vi "Floc Depth GUI.vi"(6 "Floc Depth r/w control":T2(ring), 8 "error in (no error)":errorcluster, 10 "HW.FlocEndDepthIntput":dbl[unit], 11 "Floc Depth Ref 2":T1) -> (0 "error out":errorcluster, 2 "HW.FlocEndDepth Output":dbl[unit])   [LabVIEW 2015, in "AguaClara Library.lvlib"]
uses:
  AguaClara Library.lvlib
  Floc Depth Ref.ctl
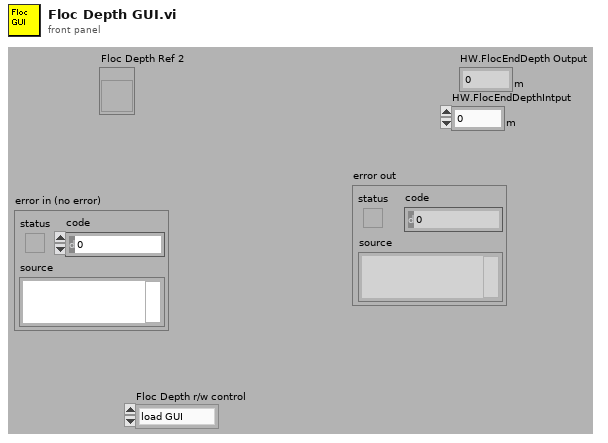
[diagram p1: front panel]
types:
  T1 = typedef "Floc Depth Ref.ctl" = refnum<vi>
  T2 = enum16{"load GUI", "write to GUI", "Update GUI", "write to basic inputs", "read from basic inputs"}
  T3 = cluster{"HW.FlocEnd":enum32{"User specified depth", "Same depth as sed tank", "Maximum depth for horizontal flow flocculator"}, "HW.FlocEndDepth":dbl[unit]}
  T4 = enum32{"User specified depth", "Same depth as sed tank", "Minimum depth for horizontal flow FLocculator"}
  T5 = enum32{"User specified depth", "Same depth as sed tank", "Maximum depth for horizontal flow flocculator"}
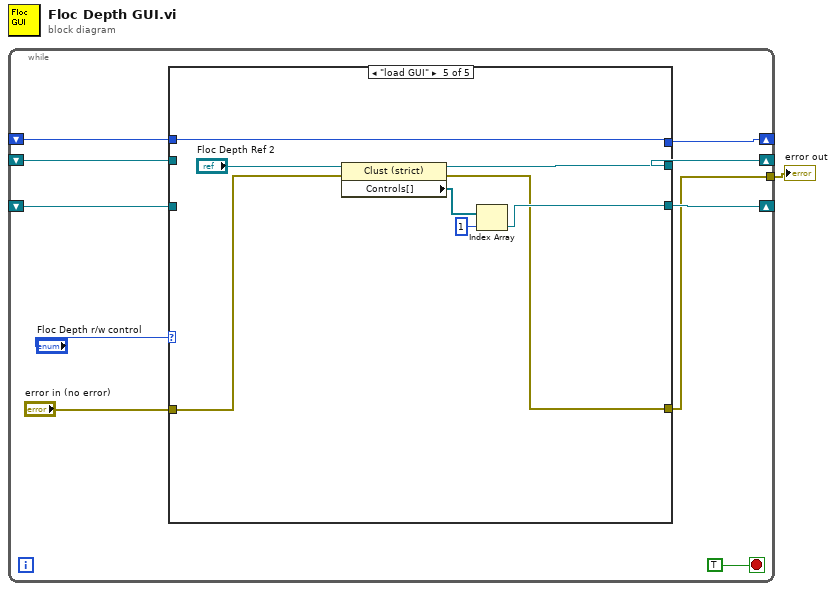
[diagram p0: block diagram]
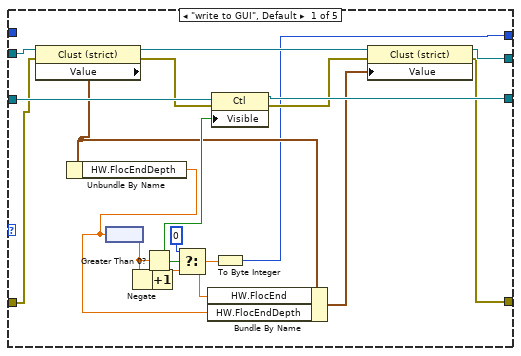
[diagram p2: hidden frame]
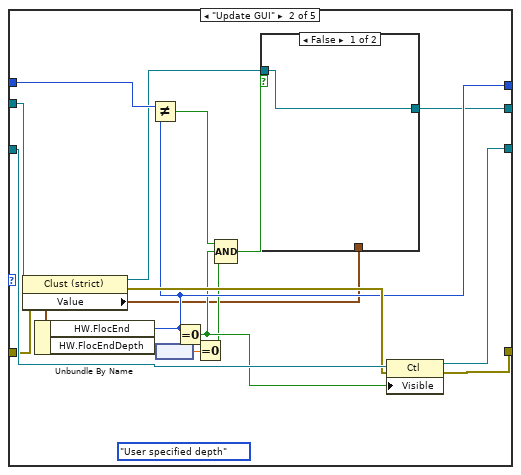
[diagram p3: hidden frame]
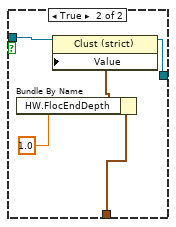
[diagram p4: hidden frame]
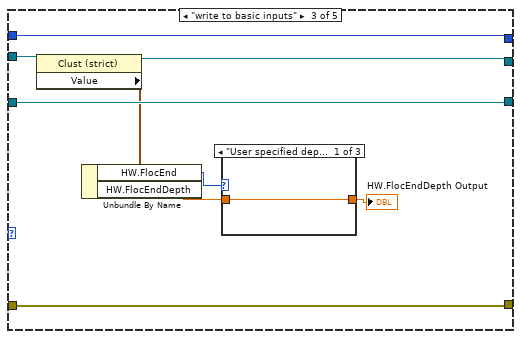
[diagram p5: hidden frame]
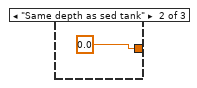
[diagram p6: hidden frame]
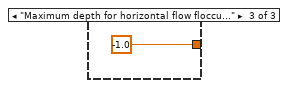
[diagram p7: hidden frame]
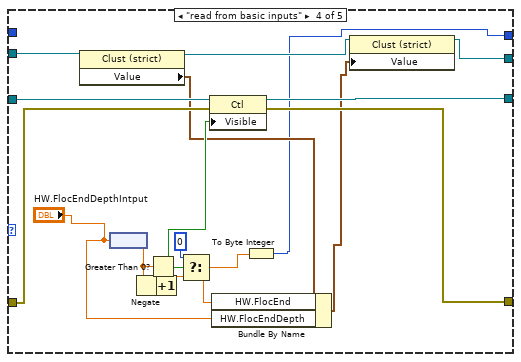
[diagram p8: hidden frame]
diagram:
  n1 = while {
    shift-right: [w9] -> _
    shift-left: _ -> [w7]
    shift-right: [w8] -> _
    shift-left: _ -> [w6]
    tunnel: [w4] -> w1
    shift-right: [w3] -> _
    shift-left: _ -> [w2]
    stop <- TRUE stop-if-true
    n2 = case shown="\"load GUI\"" "Floc Depth r/w control" {
      tunnel: w6 -> [w25 w47 w62 w76 _]
      tunnel: [w22 w31 w56 w72 w89] -> w9
      tunnel: w7 -> [w18 w44 w57 w70 _]
      tunnel: [w23 w46 w62 w75 w86] -> w8
      tunnel: [w19 w45 w61 w73 w84] -> w4
      tunnel: "error in (no error)" -> [w15 w43 w61 w74 w85]
      tunnel: [w12 w40 w54 w66 w83] -> w3
      tunnel: w2 -> [_ w41 w54 _ w83]
      frame "write to GUI", Default {
        n3 = property class="Clust (strict)"(reference=w18, error in=w15) -> (reference out=w17:T1, error out=w14:errorcluster, "Value"=w16:T3)
        n4 = Unbundle By Name(w16) -> ("HW.FlocEndDepth"=w26:dbl[unit])
        n5 = node(w26) -> (w29:dbl)
        n6 = Negate(x=w29) -> (-x=w28:dbl)
        n7 = Greater Than 0?(x=w29) -> (x > 0?=w24:bool)
        n8 = Increment(x=w28) -> (x+1=w27:dbl)
        n9 = Select(t=0, s=w24, f=w27) -> (s? t:f=w13:dbl)
        n10 = Bundle By Name(cluster=w16, "HW.FlocEnd"=w13, "HW.FlocEndDepth"=w26) -> (w21:T3)
        n11 = property class="Ctl"(reference=w25, error in=w14, "Visible"=w24) -> (reference out=w23:refnum<vi>, error out=w20:errorcluster)
        n12 = To Byte Integer(number=w13) -> (8bit integer=w12:i8)
        n13 = property class="Clust (strict)"(reference=w17, error in=w20, "Value"=w21) -> (reference out=w22:T1, error out=w19:errorcluster)
      }
      frame "Update GUI" {
        (unwired) T4."User specified depth" ("HW.FlocEnd")
        n14 = property class="Clust (strict)"(reference=w44, error in=w43) -> (reference out=w32:T1, error out=w42:errorcluster, "Value"=w33:T3)
        n15 = Unbundle By Name(w33) -> ("HW.FlocEnd"=w40:T5, "HW.FlocEndDepth"=w39:dbl[unit])
        n16 = Not Equal?(x=w41, y=w40) -> (x != y?=w37:bool)
        n17 = node(w39) -> (w38:dbl)
        n18 = Equal To 0?(x=w40) -> (x = 0?=w36:bool)
        n19 = Equal To 0?(x=w38) -> (x = 0?=w35:bool)
        n20 = Compound Arithmetic op=AND(w37, w36, w35) -> (w34:bool)
        n21 = case shown="False" w34 {
          tunnel: w32 -> [w48 w53]
          tunnel: w33 -> [_ w52]
          tunnel: [w48 w49] -> w31
          frame False {
          }
          frame True {
            n22 = Bundle By Name(cluster=w52, "HW.FlocEndDepth"=dbl[unit] 1.0) -> (w51:T3)
            n23 = property class="Clust (strict)"(reference=w53, "Value"=w51) -> (reference out=w49:T1)  [unwired: 1 in, 1 out]
          }
        }
        n24 = property class="Ctl"(reference=w47, error in=w42, "Visible"=w36) -> (reference out=w46:refnum<vi>, error out=w45:errorcluster)
      }
      frame "write to basic inputs" {
        n25 = property class="Clust (strict)"(reference=w57) -> (reference out=w56:T1, "Value"=w55:T3)  [unwired: 1 in, 1 out]
        n26 = Unbundle By Name(w55) -> ("HW.FlocEnd"=w59:T5, "HW.FlocEndDepth"=w60:dbl[unit])
        n27 = case shown="\"User specified depth\", Default" w59 {
          tunnel: [w63 dbl[unit] 0.0 ("HW.FlocEndControl") dbl[unit] -1.0 ("HW.FlocEndControl")] -> w58
          tunnel: w60 -> [w63 _ _]
          frame "User specified depth", Default {
          }
          frame "Same depth as sed tank" {
          }
          frame "Maximum depth for horizontal flow flocculator" {
          }
        }
        "HW.FlocEndDepth Output" <- w58
      }
      frame "read from basic inputs" {
        n28 = property class="Clust (strict)"(reference=w70) -> (reference out=w69:T1, "Value"=w68:T3)  [unwired: 1 in, 1 out]
        n29 = node("HW.FlocEndDepthIntput") -> (w81:dbl)
        n30 = Negate(x=w81) -> (-x=w80:dbl)
        n31 = Greater Than 0?(x=w81) -> (x > 0?=w78:bool)
        n32 = Increment(x=w80) -> (x+1=w79:dbl)
        n33 = Select(t=0, s=w78, f=w79) -> (s? t:f=w67:dbl)
        n34 = property class="Ctl"(reference=w76, error in=w74, "Visible"=w78) -> (reference out=w75:refnum<vi>, error out=w73:errorcluster)
        n35 = Bundle By Name(cluster=w68, "HW.FlocEnd"=w67, "HW.FlocEndDepth"="HW.FlocEndDepthIntput") -> (w71:T3)
        n36 = To Byte Integer(number=w67) -> (8bit integer=w66:i8)
        n37 = property class="Clust (strict)"(reference=w69, "Value"=w71) -> (reference out=w72:T1)  [unwired: 1 in, 1 out]
      }
      frame "load GUI" {
        n38 = property class="Clust (strict)"(reference="Floc Depth Ref 2", error in=w85) -> (reference out=w89:T1, error out=w84:errorcluster, "Controls[]"=w87:refnum<vi>[])
        n39 = Index Array(array=w87, index=1) -> (element=w86:refnum<vi>)
      }
    }
  }
  "error out" <- w1
